vi "updateEndTime.vi"(8 "error in (no error)":errorcluster, 11 "RfRamp in":refnum<class "RfRamp.lvclass">) -> (0 "error out":errorcluster, 3 "RfRamp out":refnum<class "RfRamp.lvclass">)   [LabVIEW 2011, in "Tools.lvlib" / "Scripting.lvlib" / "RfRamp.lvclass"]
uses:
  RfRamp.lvclass
  RfRamp.lvclass/RfRamp.ctl
  ScriptEvent.lvclass
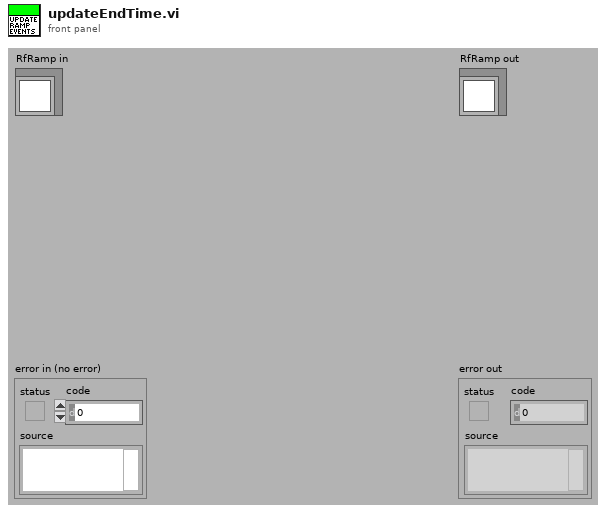
[diagram p1: front panel]
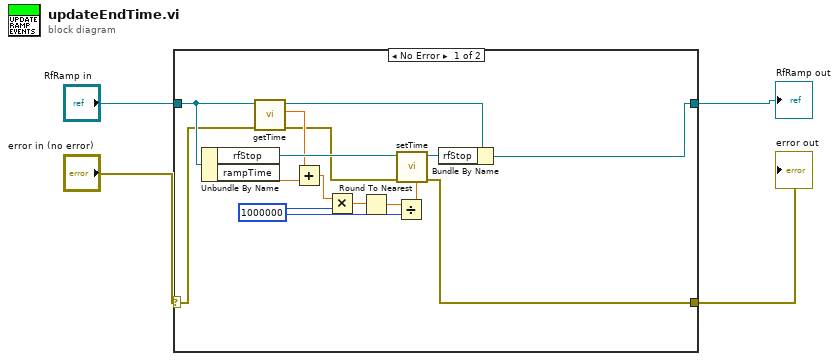
[diagram p0: block diagram]
diagram:
  n1 = case shown="No Error" "error in (no error)" {
    selector: "error in (no error)" -> [w11 w20]
    tunnel: [w12 w21] -> w4
    tunnel: "RfRamp in" -> [w18 w21]
    tunnel: [w10 w20] -> w1
    frame No Error {
      w5 = 1000000
      n2 = Unbundle By Name(w18) -> ("rfStop"=w19:refnum<class "rf.lvclass">, "rampTime"=w16:dbl)
      n3 = call "getTime.vi"("error in (no error)"=w11, "ScriptEvent.lvclass in"=w18) -> ("error out"=w15:errorcluster, "time"=w17:dbl, "ScriptEvent.lvclass out"=w14:refnum<class "RfRamp.lvclass">)  [unwired: 7 in]
      n4 = Add(x=w17, y=w16) -> (x+y=w7:dbl)
      n5 = Multiply(x=w7, y=w5) -> (x*y=w9:dbl)
      n6 = Round To Nearest(number=w9) -> (nearest integer value=w8:dbl)
      n7 = Divide(x=w8, y=w5) -> (x/y=w6:dbl)
      n8 = call "setTime.vi"("error in (no error)"=w15, "time"=w6, "ScriptEvent.lvclass in"=w19) -> ("error out"=w10:errorcluster, "ScriptEvent.lvclass out"=w13:refnum<class "rf.lvclass">)  [unwired: 7 in]
      n9 = Bundle By Name(cluster=w14, "rfStop"=w13) -> (w12:refnum<class "RfRamp.lvclass">)
    }
    frame Error {
    }
  }
  "error out" <- w1
  "RfRamp out" <- w4
